vi "GD_GWID8_S.vi"(8 "error in (no error)":errorcluster, 11 "DBlink":string="Driver={ODBC Driver 17 for SQL Server};Server=localhost\\SQLEXPRESS;Database=ZDX201;UID=labview;PWD=Dsa@54137926") -> (0 "error out":errorcluster, 2 "塗膠結果":cluster{"檢測一":string, "檢測二":string})   [LabVIEW 2019]
uses:
  <vilib>/addons/database/Connection.llb/DB Tools Open Connec (String).vi
  <vilib>/addons/database/Connection.llb/Conn Execute.vi
  <vilib>/addons/database/Recordset.llb/Rec Fetch Recordset Data (R).vi
  <vilib>/addons/database/Recordset.llb/Rec Destroy - Connection.vi
  <vilib>/addons/database/_DB Variant To Data/Database Variant To Data.xnode
  <vilib>/addons/database/NI_Database_API.lvlib
panel:
  out "Array":cluster{"檢測一":string, "檢測二":string}[](array[cluster])
  out "Command 1":string="SELECT TOP (1) [id]      \n FROM [ZDX201].[dbo].[glue_data]\n where glue_workspace_id=7 and evaluation_2 is not null\norder by id desc "
  out "Command 2":string="WHERE [id]=16"
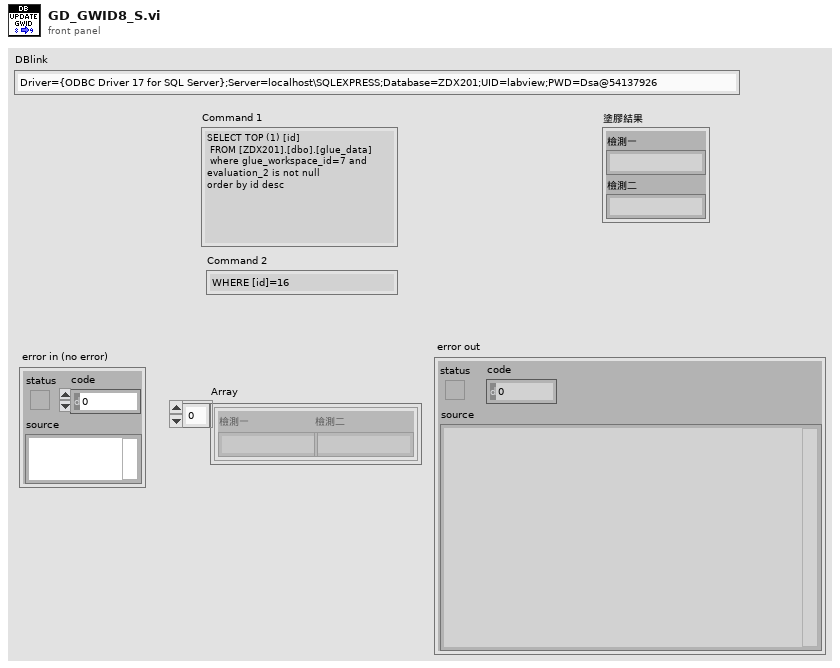
[diagram p1: front panel]
types:
  T1 = cluster{"Next GWID":i32, "update_time":timestamp}
  T2 = typedef "NI_Database_API.lvlib/Conn ObjectReference.ctl" = refnum<k1>
  T3 = typedef "NI_Database_API.lvlib/Rec ObjectReference.ctl" = refnum<k1>
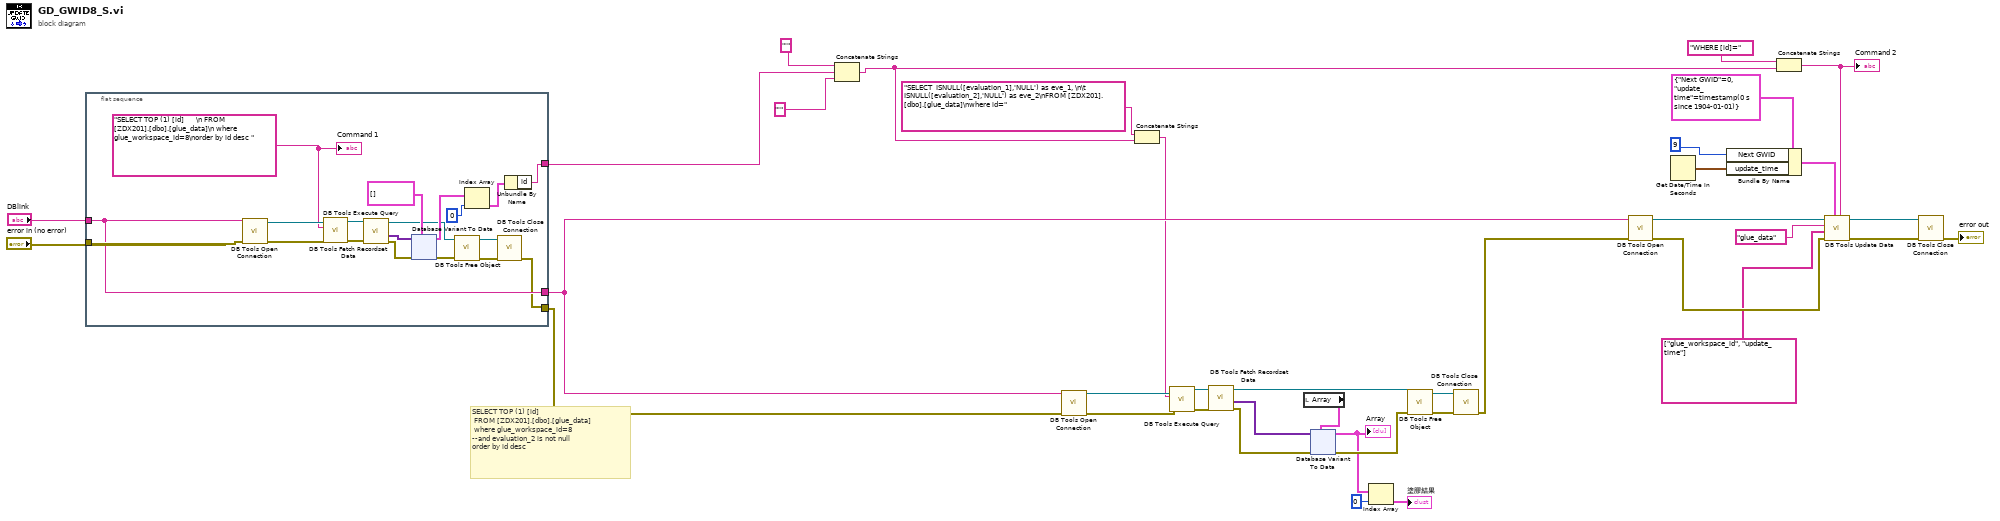
[diagram p0: block diagram]
diagram:
  # "SELECT TOP (1) [id]      \n FROM [ZDX201].[dbo].[glue_data]\n where glue_workspace_id=8 \n--and evaluation_2 is not null\norder by id desc"
  n1 = flat-sequence {
    tunnel: "DBlink" -> [w44]
    tunnel: "error in (no error)" -> [w57]
    tunnel: [w44] -> w12
    tunnel: [w41] -> w1
    tunnel: [w39] -> w11
    frame #0 {
      w40 = "SELECT TOP (1) [id]      \n FROM [ZDX201].[dbo].[glue_data]\n where glue_workspace_id=8\norder by id desc " ("SQL query")
      n2 = call-poly <vilib>:"DB Tools Open Connection.vi"("error in (no error)"=w57, "connection information"=w44) -> ("error out"=w56:errorcluster, "connection reference"=w55:T2)  [unwired: 6 in]
      n3 = call-poly <vilib>:"DB Tools Execute Query.vi"("error in (no error)"=w56, "SQL query"=w40, "connection reference"=w55) -> ("error out"=w54:errorcluster, "recordset reference"=w53:T3)  [unwired: 5 in]
      n4 = call-poly <vilib>:"DB Tools Fetch Recordset Data.vi"("error in (no error)"=w54, "recordset reference"=w53) -> ("error out"=w52:errorcluster, "recordset data"=w43:variant[][], "recordset reference out"=w45:T3)  [unwired: 3 in]
      n5 = xnode "Database Variant To Data"("database variant"=w43, "error in (no error)"=w52, "type"=cluster{"id":string}[] [] ("initialized array")) -> ("data"=w50:cluster{"id":string}[], "error out"=w46:errorcluster)
      n6 = call-poly <vilib>:"DB Tools Free Object.vi"("error in (no error)"=w46, "recordset reference"=w45) -> ("error out"=w47:errorcluster, "connection reference"=w48:T2)  [unwired: 8 in]
      n7 = Index Array(array=w50, index=0) -> (element=w42:cluster{"id":string})
      n8 = call <vilib>:"DB Tools Close Connection.vi"("error in (no error)"=w47, "connection reference"=w48) -> ("error out"=w39:errorcluster)  [unwired: 5 in]
      n9 = Unbundle By Name(w42) -> ("id"=w41:string)
      "Command 1" <- w40
    }
  }
  n10 = Concatenate Strings("'", w1, "'" ("string")) -> (w2:string)
  n11 = call-poly <vilib>:"DB Tools Open Connection.vi"("error in (no error)"=w11, "connection information"=w12) -> ("error out"=w21:errorcluster, "connection reference"=w22:T2)  [unwired: 6 in]
  n12 = Concatenate Strings("SELECT  ISNULL([evaluation_1],'NULL') as eve_1, \n\t  ISNULL([evaluation_2],'NULL') as eve_2\nFROM [ZDX201].[dbo].[glue_data]\nwhere id=" ("SQL query"), w2) -> (w10:string)
  n13 = call-poly <vilib>:"DB Tools Execute Query.vi"("error in (no error)"=w21, "SQL query"=w10, "connection reference"=w22) -> ("error out"=w20:errorcluster, "recordset reference"=w19:T3)  [unwired: 5 in]
  n14 = call-poly <vilib>:"DB Tools Fetch Recordset Data.vi"("error in (no error)"=w20, "recordset reference"=w19) -> ("error out"=w17:errorcluster, "recordset data"=w18:variant[][], "recordset reference out"=w16:T3)  [unwired: 3 in]
  n15 = local read "Array"() -> (w23:cluster{"檢測一":string, "檢測二":string}[])
  n16 = xnode "Database Variant To Data"("database variant"=w18, "error in (no error)"=w17, "type"=w23) -> ("data"=w7:cluster{"檢測一":string, "檢測二":string}[], "error out"=w15:errorcluster)
  "Array" <- w7
  n17 = Index Array(array=w7, index=0) -> (element=→"塗膠結果":cluster{"檢測一":string, "檢測二":string})
  n18 = call-poly <vilib>:"DB Tools Free Object.vi"("error in (no error)"=w15, "recordset reference"=w16) -> ("error out"=w14:errorcluster, "connection reference"=w9:T2)  [unwired: 8 in]
  n19 = call <vilib>:"DB Tools Close Connection.vi"("error in (no error)"=w14, "connection reference"=w9) -> ("error out"=w8:errorcluster)  [unwired: 5 in]
  n20 = call-poly <vilib>:"DB Tools Open Connection.vi"("error in (no error)"=w8, "connection information"=w12) -> ("error out"=w37:errorcluster, "connection reference"=w28:T2)  [unwired: 6 in]
  n21 = Get Date/Time In Seconds() -> (seconds since 1Jan1904=w24:timestamp)
  n22 = Bundle By Name(cluster=T1 {"Next GWID"=0, "update_time"=timestamp(0 s since 1904-01-01)}, "Next GWID"=9, "update_time"=w24) -> (w29:T1)
  n23 = Concatenate Strings("WHERE [id]=", w2) -> (w31:string)
  "Command 2" <- w31
  n24 = call <vilib>:"DB Tools Update Data.vi"("condition"=w31, "data"=w29, "error in (no error)"=w37, "columns"=string[] ["glue_workspace_id", "update_time"], "table"="glue_data", "connection reference"=w28) -> ("error out"=w38:errorcluster, "connection reference out"=w36:T2)  [unwired: 4 in]
  n25 = call <vilib>:"DB Tools Close Connection.vi"("error in (no error)"=w38, "connection reference"=w36) -> ("error out"=→"error out":errorcluster)  [unwired: 5 in]
